vi "SyncInputs.vi"(8 "error in (no error)":errorcluster, 10 "fpMgr in":refnum<class "LvProviderShellHelper.lvclass">, 11 "Shell in":refnum<class "LvProviderShellHelper.lvclass">) -> (0 "error out":errorcluster, 2 "fpMgr out":refnum<class "LvProviderShellHelper.lvclass">, 3 "Shell out":refnum<class "LvProviderShellHelper.lvclass">)   [LabVIEW 2019, in "LabVIEW-ProviderShell.lvlib" / "LvProviderShellHelper.lvclass"]
uses:
  LvProviderShellHelper.lvclass
  LvProviderShellHelper.lvclass/LvProviderShellHelper.ctl
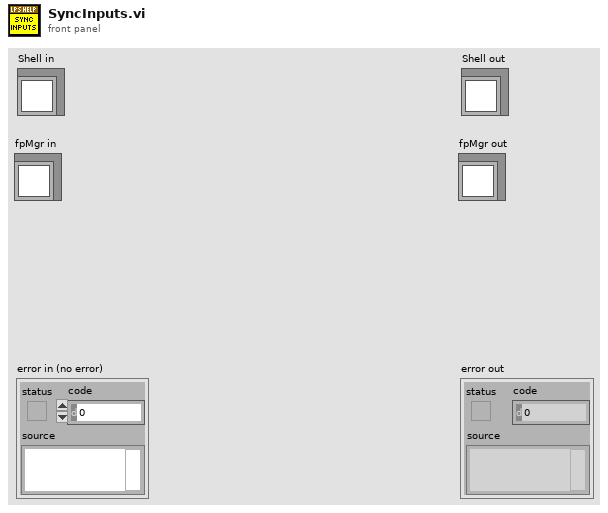
[diagram p1: front panel]
types:
  T1 = typedef "LabVIEW-ProviderShell.lvlib/LvProviderShellHelper.lvclass/def-ConnectorInfo.ctl" = cluster{"Value":variant, "Label.Text":string, "error":errorcluster, "DatatypeDescription":string, "Indicator":bool}
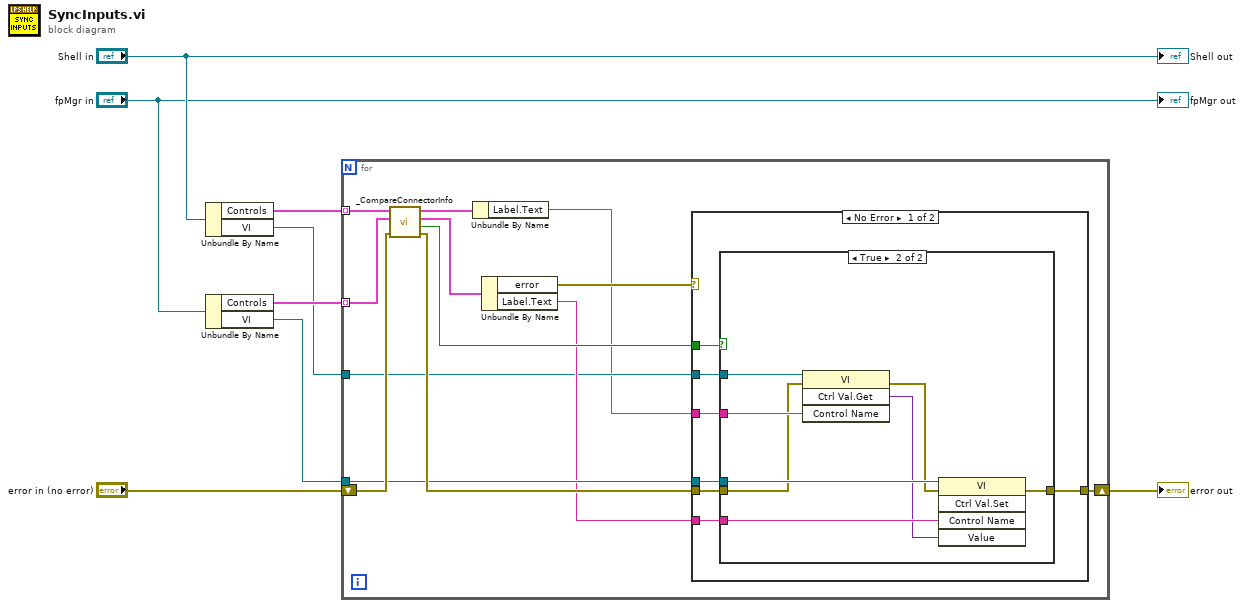
[diagram p0: block diagram]
diagram:
  n1 = Unbundle By Name("Shell in") -> ("Controls"=w6:T1[], "VI"=w1:refnum<vi>)
  n2 = Unbundle By Name("fpMgr in") -> ("Controls"=w5:T1[], "VI"=w2:refnum<vi>)
  n3 = for {
    tunnel: w6 -> [w19] mode=indexing
    tunnel: w5 -> [w18] mode=indexing
    shift-right: [w21] -> w3
    shift-left: "error in (no error)" -> [w14]
    tunnel: w2 -> [w12]
    tunnel: w1 -> [w10]
    n4 = call "_CompareConnectorInfo.vi"("error in (no error)"=w14, 10:"Cluster"=w18, 11:"Cluster"=w19) -> ("error out"=w13:errorcluster, "Matched"=w15:bool, 2:"Cluster"=w16:T1, 3:"Cluster"=w17:T1)  [unwired: 5 in]
    n5 = Unbundle By Name(w17) -> ("Label.Text"=w9:string)
    n6 = Unbundle By Name(w16) -> ("error"=w20:errorcluster, "Label.Text"=w11:string)
    n7 = case shown="No Error" w20 {
      tunnel: w12 -> [w28 _]
      tunnel: w13 -> [w27 w38]
      tunnel: [w26 w38] -> w21
      tunnel: w15 -> [w23 _]
      tunnel: w11 -> [w25 _]
      tunnel: w10 -> [w24 _]
      tunnel: w9 -> [w22 _]
      frame No Error {
        n8 = case shown="True" w23 {
          tunnel: w28 -> [_ w37]
          tunnel: w27 -> [w29 w31]
          tunnel: [w29 w36] -> w26
          tunnel: w25 -> [_ w35]
          tunnel: w24 -> [_ w34]
          tunnel: w22 -> [_ w33]
          frame False {
          }
          frame True {
            n9 = invoke class="VI" method="Ctrl Val.Get"(reference=w34, error in=w31, "Control Name"=w33) -> (error out=w30:errorcluster, "Get Control Value Variant"=w32:variant)  [unwired: 1 in, 2 out]
            n10 = invoke class="VI" method="Ctrl Val.Set"(reference=w37, error in=w30, "Control Name"=w35, "Value"=w32) -> (error out=w36:errorcluster)  [unwired: 1 in, 4 out]
          }
        }
      }
      frame Error {
      }
    }
  }
  "error out" <- w3
  "Shell out" <- "Shell in"
  "fpMgr out" <- "fpMgr in"
